vi "报警交互入队列.vi"(8 "错误输入（无错误）":errorcluster, 9 "告警内容":string, 10 "告警码":string, 11 "报警模块":string) -> (0 "错误输出":errorcluster)   [LabVIEW 2016]
panel:
  out "输出簇":T1
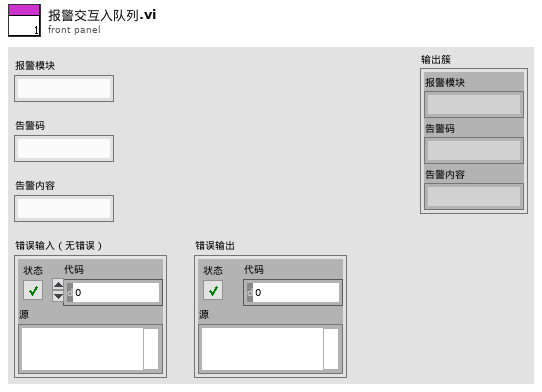
[diagram p1: front panel]
types:
  T1 = cluster{"报警模块":string, "告警码":string, "告警内容":string}
  T2 = cluster{"一级告警":string[][], "二级告警":string[][], "三级告警":string[][]}
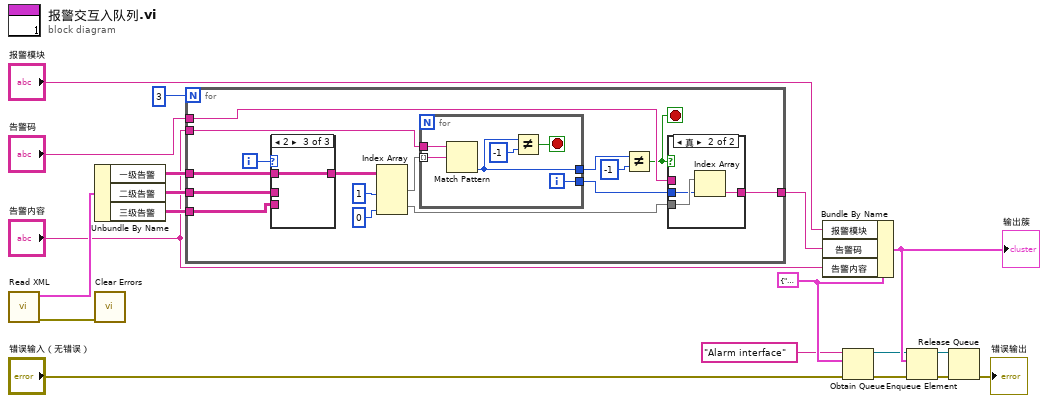
[diagram p0: block diagram]
diagram:
  w17 = T1 {"报警模块"="", "告警码"="", "告警内容"=""}
  n1 = call "Read XML.vi"() -> ("error out"=w1:errorcluster, "值"=w9:T2)  [unwired: 10 in]
  n2 = Unbundle By Name(w9) -> ("一级告警"=w8:string[][], "二级告警"=w7:string[][], "三级告警"=w6:string[][])
  n3 = call <vilib>:"Clear Errors.vi"("error in (no error)"=w1) -> ()  [unwired: 5 in, 2 out]
  n4 = for {
    N: 3 -> [_]
    tunnel: "告警内容" -> [w30]
    tunnel: "告警码" -> [w29]
    tunnel: [w26] -> w2
    tunnel: w8 -> [w25]
    tunnel: w7 -> [w24]
    tunnel: w6 -> [w23]
    i -> [w28]
    stop <- w27 stop-if-true
    n5 = case shown="2" w28 {
      tunnel: [w42 w43 w44] -> w34
      tunnel: w25 -> [_ _ w44]
      tunnel: w24 -> [_ w43 _]
      tunnel: w23 -> [w42 _ _]
      frame 0, Default {
      }
      frame 1 {
      }
      frame 2 {
      }
    }
    n6 = Index Array(array=w34, index (col) #1=1 ("禁用的索引 (列)"), index (col) #2=0 ("索引 (列)")) -> (element #1=w21:string[], element #2=w31:string[])  [unwired: 2 in]
    n7 = for {
      tunnel: w30 -> [w37]
      tunnel: [w39] -> w22
      tunnel: w21 -> [w38] mode=indexing
      tunnel: [w36] -> w20
      i -> [w36]
      stop <- w40 stop-if-true
      n8 = Match Pattern(string=w37, regular expression=w38) -> (offset past match=w39:i32)  [unwired: 1 in, 3 out]
      n9 = Not Equal?(x=w39, y=-1) -> (x != y?=w40:bool)
    }
    n10 = Not Equal?(x=w22, y=-1) -> (x != y?=w27:bool)
    n11 = case shown="真" w27 {
      tunnel: w31 -> [_ w48]
      tunnel: w20 -> [_ w47]
      tunnel: [w45 w46] -> w26
      tunnel: w29 -> [w45 _]
      frame False {
      }
      frame True {
        n12 = Index Array(array=w48, index=w47) -> (element=w46:string)
      }
    }
  }
  n13 = Bundle By Name(cluster=w17, "报警模块"="报警模块", "告警码"=w2, "告警内容"="告警内容") -> (w18:T1)
  "输出簇" <- w18
  n14 = Obtain Queue(name (unnamed)="Alarm interface" ("名称（未命名）"), element data type=w17, error in (no error)="错误输入（无错误）") -> (queue out=w13:refnum<queue>, error out=w14:errorcluster)  [unwired: 2 in, 1 out]
  n15 = Enqueue Element(queue=w13, element=w18, error in (no error)=w14) -> (queue out=w15:refnum<queue>, error out=w16:errorcluster)  [unwired: 1 in, 1 out]
  n16 = Release Queue(queue=w15, error in (no error)=w16) -> (error out=→"错误输出":errorcluster)  [unwired: 1 in, 2 out]
